vi "ConvertVItoHTML.vi"(0 "vi name":string) -> (1 "Htm log name":string, 2 "Server Name":string)   [LabVIEW 2012]
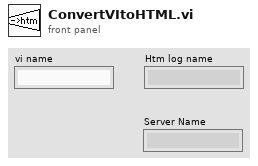
[diagram p1: front panel]
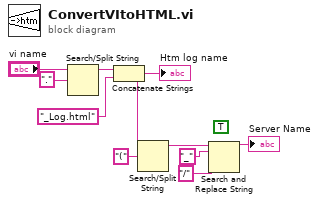
[diagram p0: block diagram]
diagram:
  (unwired) TRUE ("replace all? (F)")
  n1 = Search/Split String(string="vi name", search string/char (-)=".") -> (substring before match=w8:string)  [unwired: 1 in, 2 out]
  n2 = Concatenate Strings(w8, "_Log.html" ("string")) -> (w2:string)
  "Htm log name" <- w2
  n3 = Search/Split String(string=w2, search string/char (-)="(") -> (substring before match=w5:string)  [unwired: 1 in, 2 out]
  n4 = Search and Replace String(input string=w5, search string="_", replace string="/" ("replace string (\"\")")) -> (result string=→"Server Name":string)  [unwired: 5 in, 3 out]
